vi "ideal_gas_heat_capacity_humid_air_2024.vi"(7 "molar fraction of water vapor":dbl, 9 "Temperature [K]":dbl=293.15 format="%.4g", 11 "Type of air":i32(listbox)=4, 13 "CO2 content (ppm)":dbl=500.0) -> (0 "Cp0/R water":dbl=4.037070056851789, 1 "Cp0 water [J / Kmol]":dbl=33.566068001274076, 2 "Cp0/R humid air":dbl=3.499501241139648, 3 "Cp0/R dry air":dbl=3.499501241139648, 4 "Cv0 water [J / Kmol]":dbl=25.251605401274077, 5 "Cv0 dry [J / Kmol]":dbl=20.782009588109183, 8 "Gamma0 dry":dbl=1.400079817341499, 10 "Gamma0 water":dbl=1.329264712792498, 12 "Cp0 dry [J / Kmol]":dbl=29.096472188109185, 15 "Gamma0 humid air":dbl=1.4000798173414988)   [LabVIEW 2016]
uses:
  2022/SOS_Global_2022.vi
panel:
  out "CO2 content / ppm":dbl=500.0
  out "rel. differs from 1.400 by / ppm":dbl=57.012386784904834
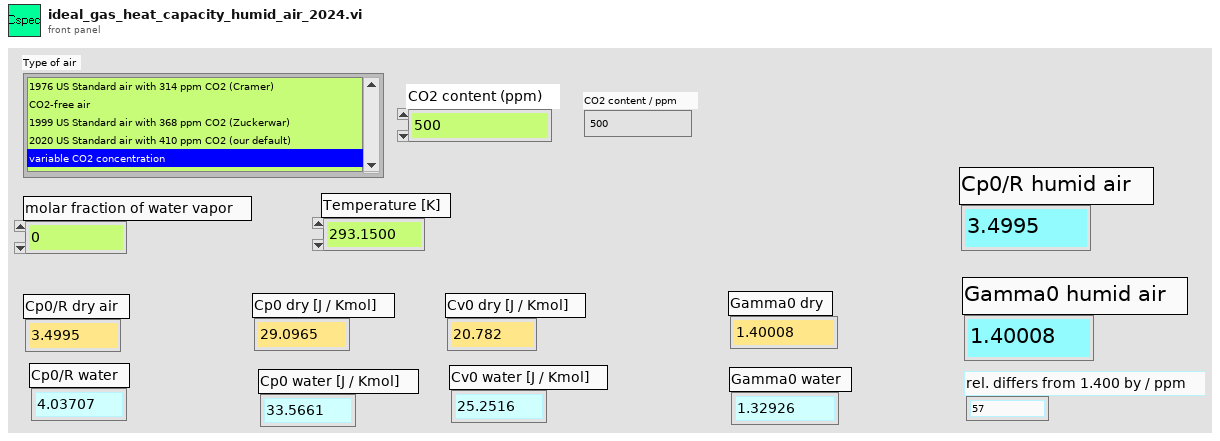
[diagram p1: front panel]
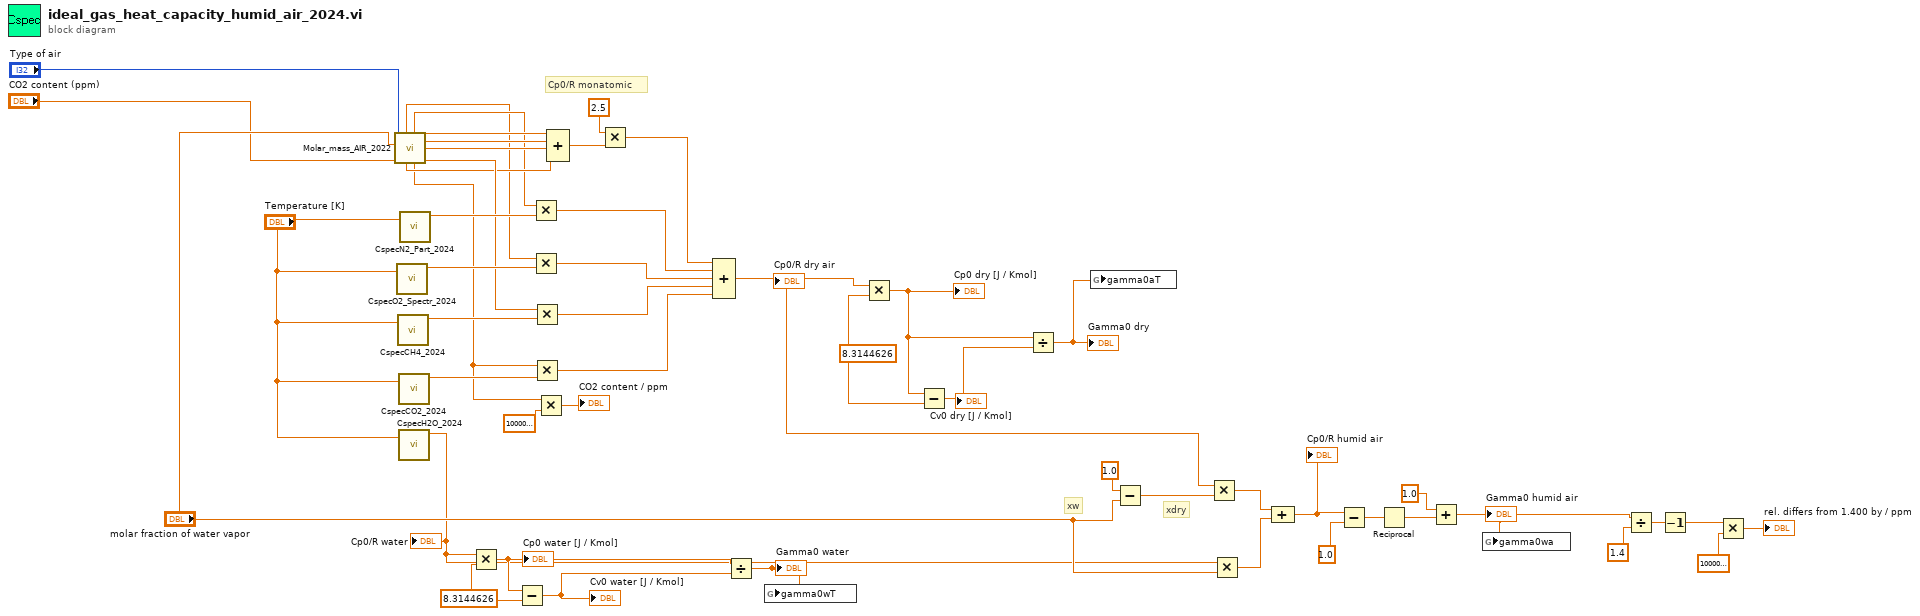
[diagram p0: block diagram]
diagram:
  w17 = 8.3144626
  w37 = 8.3144626
  # "xdry"
  # "xw"
  # "Cp0/R monatomic"
  n1 = call "Molar_mass_AIR_2022.vi"("CO2 content (ppm)"="CO2 content (ppm)", "xw molar fraction of water vapor"="molar fraction of water vapor", "Type of air"="Type of air") -> ("xCH4"=w47:dbl, "xKr"=w43:dbl, "xHe"=w44:dbl, "xNe"=w45:dbl, "xCO2"=w2:dbl, "xN2"=w34:dbl, "xAr"=w36:dbl, "xO2"=w33:dbl)  [unwired: 1 out]
  n2 = call "CspecO2_Spectr_2024.vi"("Temperature [K]"="Temperature [K]") -> ("Cp0/R O2"=w48:dbl)  [unwired: 4 out]
  n3 = call "CspecCH4_2024.vi"("Temperature [K]"="Temperature [K]") -> ("Cp0/R CH4"=w32:dbl)  [unwired: 4 out]
  n4 = call "CspecCO2_2024.vi"("Temperature [K]"="Temperature [K]") -> ("Cp0/R CO2"=w31:dbl)  [unwired: 4 out]
  n5 = call "CspecH2O_2024.vi"("Temperature [K]"="Temperature [K]") -> ("Cp0/R water"=w14:dbl)  [unwired: 4 out]
  "Cp0/R water" <- w14
  n6 = call "CspecN2_Part_2024.vi"("Temperature [K]"="Temperature [K]") -> ("Cp0/R N2"=w49:dbl)  [unwired: 4 out]
  n7 = Multiply(x=w14, y=w17) -> (x*y=w16:dbl)
  "Cp0 water [J / Kmol]" <- w16
  n8 = Subtract(x=w16, y=w17) -> (x-y=w15:dbl)
  "Cv0 water [J / Kmol]" <- w15
  n9 = Multiply(x=w34, y=w49) -> (x*y=w41:dbl)
  n10 = Multiply(x=w33, y=w48) -> (x*y=w40:dbl)
  n11 = Multiply(x=w47, y=w32) -> (x*y=w39:dbl)
  n12 = Multiply(x=w2, y=w31) -> (x*y=w38:dbl)
  n13 = Multiply(x=w2, y=1000000.0) -> (x*y=→"CO2 content / ppm":dbl)
  n14 = Compound Arithmetic op=ADD(w45, w44, w43, w36) -> (w35:dbl)
  n15 = Multiply(x=2.5, y=w35) -> (x*y=w42:dbl)
  n16 = Compound Arithmetic op=ADD(w42, w41, w40, w39, w38) -> (w23:dbl)
  "Cp0/R dry air" <- w23
  n17 = Divide(x=w16, y=w15) -> (x/y=w24:dbl)
  "Gamma0 water" <- w24
  n18 = global write "SOS_Global_2022.vi" "gamma0wT"(w24) -> ()
  n19 = Multiply(x=w23, y=w37) -> (x*y=w19:dbl)
  "Cp0 dry [J / Kmol]" <- w19
  n20 = Subtract(x=w19, y=w37) -> (x-y=w18:dbl)
  "Cv0 dry [J / Kmol]" <- w18
  n21 = Divide(x=w19, y=w18) -> (x/y=w20:dbl)
  "Gamma0 dry" <- w20
  n22 = global write "SOS_Global_2022.vi" "gamma0aT"(w20) -> ()
  n23 = Subtract(x=1.0, y="molar fraction of water vapor") -> (x-y=w29:dbl)
  n24 = Multiply(x=w23, y=w29) -> (x*y=w13:dbl)
  n25 = Multiply(x=w14, y="molar fraction of water vapor") -> (x*y=w28:dbl)
  n26 = Compound Arithmetic op=ADD(w13, w28) -> (w4:dbl)
  "Cp0/R humid air" <- w4
  n27 = Subtract(x=w4, y=1.0) -> (x-y=w12:dbl)
  n28 = Reciprocal(x=w12) -> (1/x=w11:dbl)
  n29 = Add(x=1.0, y=w11) -> (x+y=w10:dbl)
  "Gamma0 humid air" <- w10
  n30 = global write "SOS_Global_2022.vi" "gamma0wa"(w10) -> ()
  n31 = Divide(x=w10, y=1.4) -> (x/y=w8:dbl)
  n32 = Decrement(x=w8) -> (x-1=w7:dbl)
  n33 = Multiply(x=w7, y=1000000.0) -> (x*y=→"rel. differs from 1.400 by / ppm":dbl)
